vi "test Endpoint Configurations.vi"(8 "error in (no error)":errorcluster, 11 "TestCase in":refnum<class "SLSC Switch Scripting Unit Tests.lvclass">) -> (0 "error out":errorcluster, 3 "TestCase out":refnum<class "SLSC Switch Scripting Unit Tests.lvclass">)   [LabVIEW 2017, in "SLSC Switch Scripting Unit Tests.lvclass"]
uses:
  SLSC Switch Scripting Unit Tests.lvclass
  Shared/Endpoint Configuration Cluster.ctl
  Shared/Endpoint Configuration Enum.ctl
  SLSC Switch Scripting Unit Tests.lvclass/SLSC Switch Scripting Unit Tests.ctl
  <vilib>/addons/_JKI Toolkits/VI Tester/TestCase.llb/TestCase.lvclass
  SLSC Switch Scripting.lvlib
  Shared/SLSC Switch Shared.lvlib
  C:/Program Files (x86)/National Instruments/LabVIEW 2017/vi.lib/addons/_JKI Toolkits/VI Tester/TestCase.llb/TestCase.lvclass
panel:
  in  "Save?":bool
  out "Output Filename":string
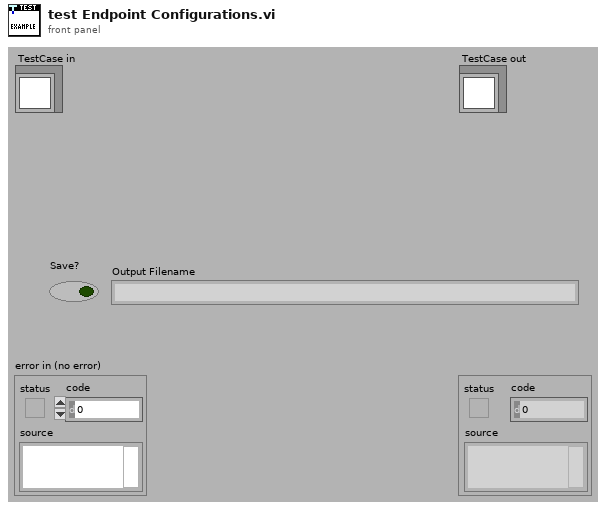
[diagram p1: front panel]
types:
  T1 = typedef "SLSC Switch Shared.lvlib/Endpoint Configuration Cluster.ctl" = cluster{"Endpoint":string, "Configuration":T2}
  T2 = typedef "SLSC Switch Shared.lvlib/Endpoint Configuration Enum.ctl" = enum16{"Load", "Source", "Configuration"}
  T3 = typedef "Custom Device API.lvlib/Custom Device Item Ref.ctl" = u64
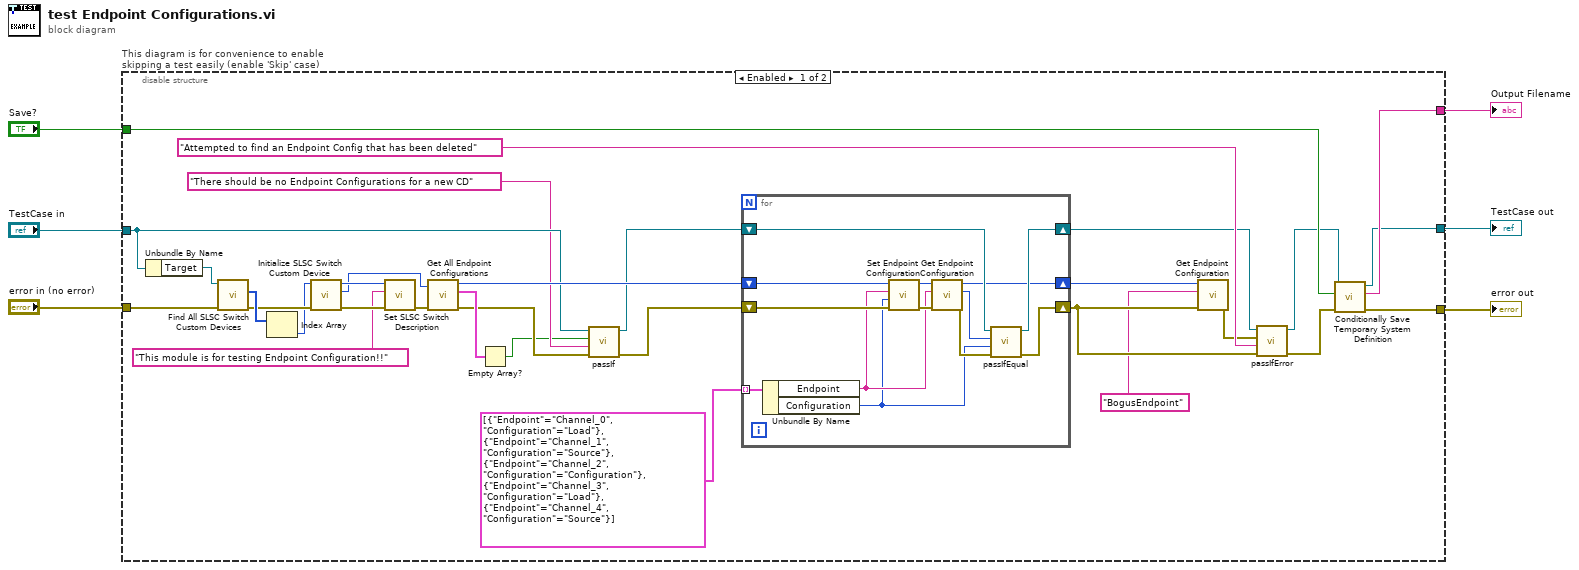
[diagram p0: block diagram]
diagram:
  n1 = disable-structure "This diagram is for convenience to enable skipping a test easily (enable 'Skip' case)" shown="Enabled" {
    disable-tunnel: "TestCase in" -> [w22 w54]
    disable-tunnel: [w35 w52] -> w3
    disable-tunnel: [w36 w53] -> w5
    disable-tunnel: "error in (no error)" -> [w29 w51]
    disable-tunnel: [w37 _] -> w2
    disable-tunnel: "Save?" -> [w34 _]
    frame Enabled {
      n2 = Unbundle By Name(w22) -> ("Target"=w30:refnum<k24>)
      n3 = call "Find All SLSC Switch Custom Devices.vi"("error in (no error)"=w29, "Target in"=w30) -> ("error out"=w32:errorcluster, "SLSC Switch Custom Device Ref IDs"=w33:T3[])  [unwired: 7 in, 1 out]
      n4 = Index Array(array=w33) -> (element=w31:T3)  [unwired: 1 in]
      n5 = call "Initialize SLSC Switch Custom Device.vi"("error in (no error)"=w32, "SLSC Switch Custom Device Ref in"=w31) -> ("error out"=w27:errorcluster, "Endpoint Configuration Section Ref"=w25:T3, "SLSC Switch Custom Device Ref out"=w28:T3)  [unwired: 7 in]
      n6 = call "Set SLSC Switch Description.vi"("error in (no error)"=w27, "Description"="This module is for testing Endpoint Configuration!!", "SLSC Switch Custom Device Ref in"=w28) -> ("error out"=w18:errorcluster)  [unwired: 7 in, 1 out]
      n7 = call "Get All Endpoint Configurations.vi"("error in (no error)"=w18, "Endpoint Configuration Section Ref in"=w25) -> ("error out"=w10:errorcluster, "All Endpoint Configurations"=w23:T1[], "Endpoint Configuration Section Ref out"=w24:T3)  [unwired: 7 in]
      n8 = Empty Array?(array=w23) -> (empty?=w8:bool)
      n9 = call-dynamic "passIf.vi"("error in (no error)"=w10, "message (\"\")"="There should be no Endpoint Configurations for a new CD" ("message (\"\")"), "pass"=w8, "TestCase in"=w22) -> ("error out"=w19:errorcluster, "TestCase out"=w21:refnum<class "SLSC Switch Scripting Unit Tests.lvclass">)  [unwired: 6 in]
      n10 = for {
        shift-right: [w43] -> w16
        shift-left: w19 -> [w49]
        shift-right: [w45] -> w14
        shift-left: w21 -> [w46]
        shift-right: [w42] -> w17
        shift-left: w24 -> [w50]
        tunnel: T1[] [{"Endpoint"="Channel_0", "Configuration"=enum."Load"}, {"Endpoint"="Channel_1", "Configuration"=enum."Source"}, {"Endpoint"="Channel_2", "Configuration"=enum."Configuration"}, {"Endpoint"="Channel_3", "Configuration"=enum."Load"}, {"Endpoint"="Channel_4", "Configuration"=enum."Source"}] ("Array") -> [w40] mode=indexing
        n11 = Unbundle By Name(w40) -> ("Endpoint"=w39:string, "Configuration"=w38:T2)
        n12 = call "Set Endpoint Configuration.vi"("error in (no error)"=w49, "Configuration Type"=w38, "Endpoint"=w39, "Endpoint Configuration Section Ref in"=w50) -> ("error out"=w47:errorcluster, "Endpoint Configuration Section Ref out"=w48:T3)  [unwired: 6 in]
        n13 = call "Get Endpoint Configuration.vi"("error in (no error)"=w47, "Endpoint"=w39, "Endpoint Configuration Section Ref in"=w48) -> ("error out"=w44:errorcluster, "Configuration Type"=w41:T2, "Endpoint Configuration Section Ref out"=w42:T3)  [unwired: 6 in]
        n14 = call-dynamic "passIfEqual.vi"("error in (no error)"=w44, "y"=w38, "x"=w41, "TestCase in"=w46) -> ("error out"=w43:errorcluster, "TestCase out"=w45:refnum<class "SLSC Switch Scripting Unit Tests.lvclass">)  [unwired: 6 in]
      }
      n15 = call "Get Endpoint Configuration.vi"("error in (no error)"=w16, "Endpoint"="BogusEndpoint", "Endpoint Configuration Section Ref in"=w17) -> ("error out"=w12:errorcluster)  [unwired: 6 in, 2 out]
      n16 = call-dynamic "passIfError.vi"("error in (no error)"=w16, "task (\"\")"="Attempted to find an Endpoint Config that has been deleted" ("message (\"\")"), "error"=w12, "TestCase in"=w14) -> ("error out"=w11:errorcluster, "TestCase out"=w13:refnum<class "SLSC Switch Scripting Unit Tests.lvclass">)  [unwired: 6 in]
      n17 = call "Conditionally Save Temporary System Definition.vi"("error in (no error)"=w11, "Save?"=w34, "Test Case"=w13) -> ("error out"=w36:errorcluster, "filename"=w37:string, "Test Case"=w35:refnum<class "SLSC Switch Scripting Unit Tests.lvclass">)  [unwired: 6 in]
    }
    frame Disabled {
      # "skip test result while test is under development"
      n18 = call <vilib>:"skip.vi"("error in (no error)"=w51, "TestCase in"=w54) -> ("error out"=w53:errorcluster, "TestCase out"=w52:refnum<class "SLSC Switch Scripting Unit Tests.lvclass">)  [unwired: 8 in]
    }
  }
  "error out" <- w5
  "TestCase out" <- w3
  "Output Filename" <- w2
